vi "LP_Intro.vi"   [LabVIEW 2012]
uses:
  SubVIs/LVPresent_Globals.vi
panel:
  # "Click the arrow to start the presentation."
  # "LilyPad: Getting Started\n\nThe goal of this book is to get you started in LabVIEW with the LilyPad - you will need 1 LilyPad - please connect it up."
  # "Vibrator"
  # "Temperature Sensor"
  # "Light Sensor"
  # "RGB LEDs"
  # "Buzzer"
  # "Button"
  # "Switch"
  # "LEDs"
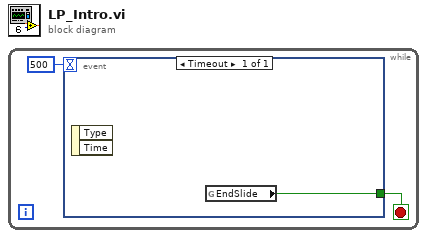
[diagram p0: block diagram]
diagram:
  n1 = while {
    stop <- w2 stop-if-true
    n2 = event shown="[0] Timeout" {
      selector: _ -> [_]
      dyn-events: _ -> [_]
      timeout: 500 -> [_]
      tunnel: [w3] -> w2
      event Timeout {
        n3 = event-data() -> ()  [unwired: 1 in, 2 out]
        n4 = global read "LVPresent_Globals.vi" "EndSlide"() -> (w3:bool)
      }
    }
  }
